vi "Item_OnCommand.vi"(10 "Command ID":string, 11 "Object":T1) -> ()   [LabVIEW 2018, in "LVClassByRef.lvlib"]
uses:
  <resource>/Framework/Providers/LVClassByRef/LVClassByRef.lvlib
  <resource>/Framework/Providers/API/ItemRef.ctl
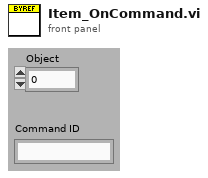
[diagram p1: front panel]
types:
  T1 = typedef "ItemRef.ctl" = u64
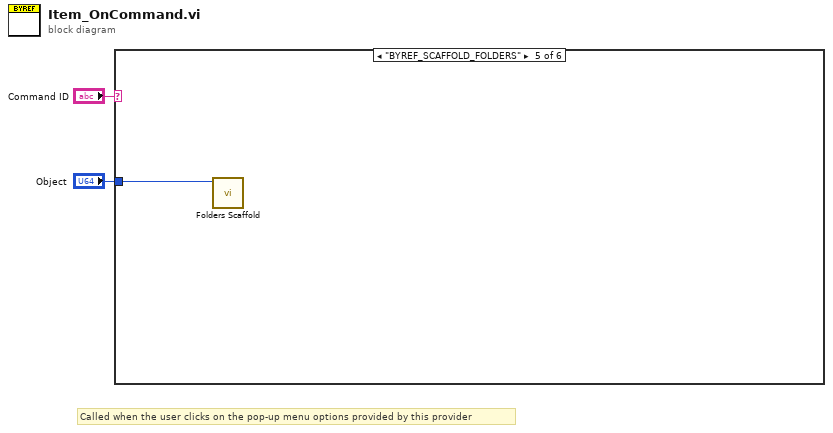
[diagram p0: block diagram]
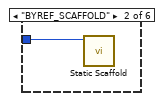
[diagram p3: hidden frame]
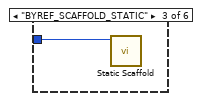
[diagram p4: hidden frame]
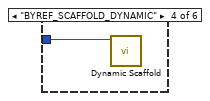
[diagram p5: hidden frame]
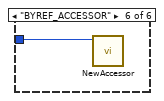
[diagram p6: hidden frame]
diagram:
  # "Called when the user clicks on the pop-up menu options provided by this provider"
  n1 = case shown="\"BYREF_SCAFFOLD_FOLDERS\"" "Command ID" {
    tunnel: "Object" -> [_ w3 w4 w5 w6 w7]
    frame Default {
    }
    frame "BYREF_SCAFFOLD" {
      n2 = call <resource>:"Static Scaffold.vi"("Object"=w3) -> ()  [unwired: 11 in]
    }
    frame "BYREF_SCAFFOLD_STATIC" {
      n3 = call <resource>:"Static Scaffold.vi"("Object"=w4) -> ()  [unwired: 11 in]
    }
    frame "BYREF_SCAFFOLD_DYNAMIC" {
      n4 = call <resource>:"Dynamic Scaffold.vi"("Object"=w5) -> ()  [unwired: 11 in]
    }
    frame "BYREF_SCAFFOLD_FOLDERS" {
      n5 = call <resource>:"Folders Scaffold.vi"("Object"=w6) -> ()  [unwired: 11 in]
    }
    frame "BYREF_ACCESSOR" {
      n6 = call <resource>:"NewAccessor.vi"("Object"=w7) -> ()  [unwired: 11 in]
    }
  }
